vi "固件升级对话框.vi"() -> ()   [LabVIEW 2016, in "斯坦道通用流路CODmn.lvlib"]
uses:
  <vilib>/Utility/miscctls.llb/LVPointTypeDef.ctl
panel:
  in  "备份参数":bool
  in  "恢复参数":bool
  in  "关闭":bool
  in  "固件升级":bool
  in  "固件状态":bool
  out "结果字符串":string
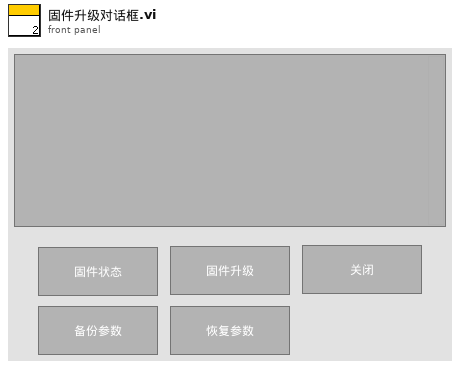
[diagram p1: front panel]
types:
  T1 = typedef "LVPointTypeDef.ctl" = cluster{"Horizontal":i16, "Vertical":i16}
  T2 = typedef "操作日志字段定义.ctl" = cluster{"时间":timestamp, "参数":string, "日志信息":string, "流程参数":string}
  T3 = cluster{"Value":u16, i32, i32, "公式":cluster{"X^2":dbl, "X":dbl, "b":dbl}, "error out":errorcluster}[][][]
  T4 = cluster{"Value":u16, "量程参数读取":cluster{"测量精度":u16, "检出限":dbl, "上限":dbl, "下限":dbl, "阈值（低->高）":dbl, "阈值（高->低）":dbl, "稀释度":dbl}, "error out":errorcluster}[]
  T5 = cluster{"试剂容量":cluster{"V1":sgl, "V2":sgl, "V3":sgl, "V4":sgl, "V5":sgl, "V6":sgl, "V7":sgl, "V8":sgl, "V9":sgl, "V10":sgl, "V11":sgl, "V12":sgl, "V9-1":sgl, "V9-2":sgl}, "error out":errorcluster}
  T6 = typedef "SingleStepTestV3.lvlib/SingleStepTestV3.lvclass/仪器版本.ctl" = enum16{"A版", "B版", "A1版"}
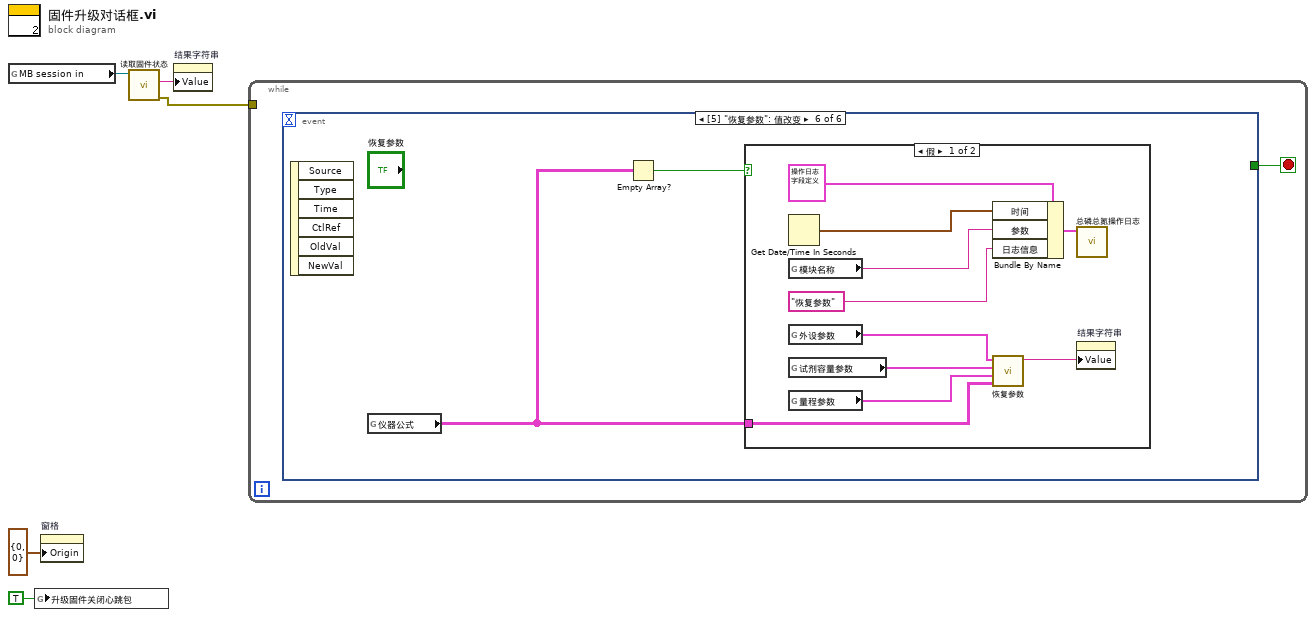
[diagram p0: block diagram]
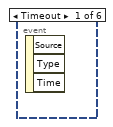
[diagram p2: hidden frame]
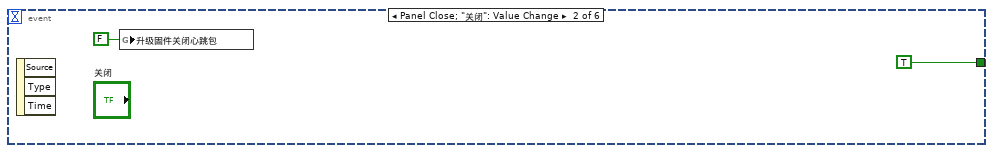
[diagram p3: hidden frame]
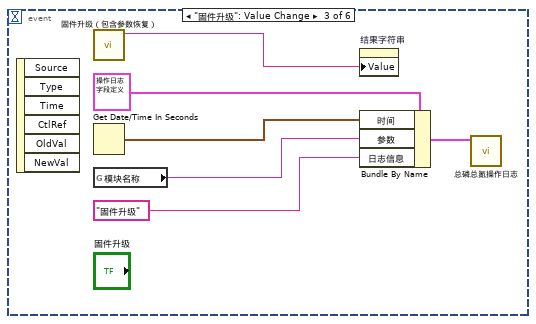
[diagram p4: hidden frame]
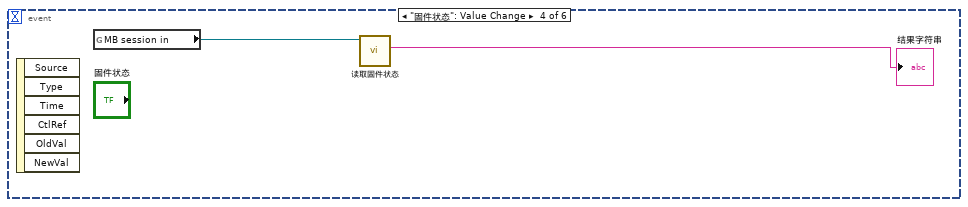
[diagram p5: hidden frame]
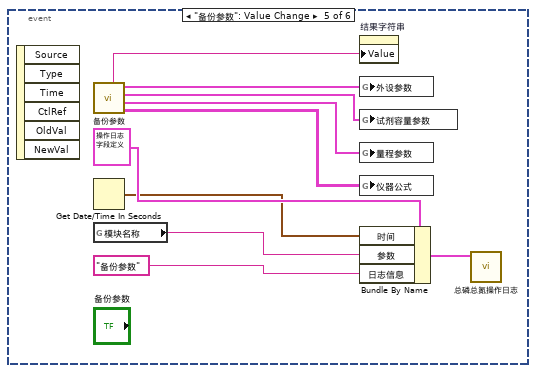
[diagram p6: hidden frame]
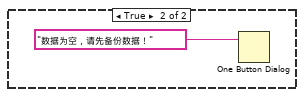
[diagram p7: hidden frame]
diagram:
  n1 = global read "VAR总磷总氮全局变量.vi" "MB session in"() -> (w4:refnum<class "MB_Master.lvclass">)
  n2 = global write "VAR总磷总氮全局变量.vi" "升级固件关闭心跳包"(TRUE ("升级固件关闭心跳包")) -> ()
  n3 = property on="窗格" class="Pane"("Origin"=T1 {"Horizontal"=0, "Vertical"=0} ("原点")) -> ()  [unwired: 2 in, 2 out]
  n4 = call "读取固件状态.vi"("MB session in"=w4) -> ("error out"=w3:errorcluster, "结果字符串"=w1:string)  [unwired: 7 in, 2 out]
  n5 = property on="结果字符串" class="Str"("Value"=w1) -> ()  [unwired: 2 in, 2 out]
  n6 = while {
    tunnel: w3 -> [_]
    stop <- w6 stop-if-true
    n7 = event shown="[5] \"恢复参数\": 值改变" {
      selector: _ -> [_ _ _ _ _ _]
      dyn-events: _ -> [_ _ _ _ _ _]
      timeout: _ -> [_ _ _ _ _ _]
      tunnel: [_ TRUE _ _ _ _] -> w6
      event Timeout {
        n8 = event-data() -> ()  [unwired: 1 in, 3 out]
      }
      event Panel Close; "关闭": Value Change {
        n9 = event-data() -> ()  [unwired: 1 in, 3 out]
        n10 = global write "VAR总磷总氮全局变量.vi" "升级固件关闭心跳包"(FALSE ("升级固件关闭心跳包")) -> ()
      }
      event "固件升级": Value Change {
        n11 = event-data() -> ()  [unwired: 1 in, 6 out]
        n12 = call "固件升级（包含参数恢复）.vi"() -> ("结果字符串"=w14:string)  [unwired: 11 in]
        n13 = Get Date/Time In Seconds() -> (seconds since 1Jan1904=w11:timestamp)
        n14 = global read "VAR总磷总氮全局变量.vi" "模块名称"() -> (w9:string)
        n15 = property on="结果字符串" class="Str"("Value"=w14) -> ()  [unwired: 2 in, 2 out]
        n16 = Bundle By Name(cluster=T2 {"时间"=timestamp(0 s since 1904-01-01), "参数"="", "日志信息"="", "流程参数"=""} ("data in"), "时间"=w11, "参数"=w9, "日志信息"="固件升级") -> (w12:T2)
        n17 = call "总磷总氮操作日志.vi"("data in"=w12) -> ()  [unwired: 10 in, 1 out]
      }
      event "固件状态": Value Change {
        n18 = event-data() -> ()  [unwired: 1 in, 6 out]
        n19 = global read "VAR总磷总氮全局变量.vi" "MB session in"() -> (w15:refnum<class "MB_Master.lvclass">)
        n20 = call "读取固件状态.vi"("MB session in"=w15) -> ("结果字符串"=→"结果字符串":string)  [unwired: 7 in, 3 out]
      }
      event "备份参数": Value Change {
        n21 = event-data() -> ()  [unwired: 1 in, 6 out]
        n22 = call "备份参数.vi"() -> ("仪器公式"=w23:T3, "量程参数"=w24:T4, "试剂容量参数"=w25:T5, "外设参数"=w26:cluster{"仪器版本":T6, "error out":errorcluster}, "备份结果"=w22:string)  [unwired: 7 in]
        n23 = Get Date/Time In Seconds() -> (seconds since 1Jan1904=w19:timestamp)
        n24 = global read "VAR总磷总氮全局变量.vi" "模块名称"() -> (w17:string)
        n25 = property on="结果字符串" class="Str"("Value"=w22) -> ()  [unwired: 2 in, 2 out]
        n26 = global write "VAR总磷总氮全局变量.vi" "外设参数"(w26) -> ()
        n27 = global write "VAR总磷总氮全局变量.vi" "试剂容量参数"(w25) -> ()
        n28 = global write "VAR总磷总氮全局变量.vi" "量程参数"(w24) -> ()
        n29 = global write "VAR总磷总氮全局变量.vi" "仪器公式"(w23) -> ()
        n30 = Bundle By Name(cluster=T2 {"时间"=timestamp(0 s since 1904-01-01), "参数"="", "日志信息"="", "流程参数"=""} ("data in"), "时间"=w19, "参数"=w17, "日志信息"="备份参数") -> (w20:T2)
        n31 = call "总磷总氮操作日志.vi"("data in"=w20) -> ()  [unwired: 10 in, 1 out]
      }
      event "恢复参数": Value Change {
        n32 = event-data() -> ()  [unwired: 1 in, 6 out]
        n33 = global read "VAR总磷总氮全局变量.vi" "仪器公式"() -> (w28:T3)
        n34 = Empty Array?(array=w28) -> (empty?=w27:bool)
        n35 = case shown="假" w27 {
          tunnel: w28 -> [w34 _]
          frame False {
            n36 = Get Date/Time In Seconds() -> (seconds since 1Jan1904=w31:timestamp)
            n37 = global read "VAR总磷总氮全局变量.vi" "模块名称"() -> (w29:string)
            n38 = global read "VAR总磷总氮全局变量.vi" "外设参数"() -> (w36:cluster{"仪器版本":T6, "error out":errorcluster})
            n39 = global read "VAR总磷总氮全局变量.vi" "试剂容量参数"() -> (w37:T5)
            n40 = global read "VAR总磷总氮全局变量.vi" "量程参数"() -> (w38:T4)
            n41 = Bundle By Name(cluster=T2 {"时间"=timestamp(0 s since 1904-01-01), "参数"="", "日志信息"="", "流程参数"=""} ("data in"), "时间"=w31, "参数"=w29, "日志信息"="恢复参数") -> (w32:T2)
            n42 = call "恢复参数.vi"("仪器公式"=w34, "量程参数"=w38, "试剂容量参数"=w37, "外设参数"=w36) -> ("恢复结果"=w35:string)  [unwired: 7 in]
            n43 = call "总磷总氮操作日志.vi"("data in"=w32) -> ()  [unwired: 10 in, 1 out]
            n44 = property on="结果字符串" class="Str"("Value"=w35) -> ()  [unwired: 2 in, 2 out]
          }
          frame True {
            n45 = One Button Dialog(message="数据为空，请先备份数据！" ("消息")) -> ()  [unwired: 1 in, 1 out]
          }
        }
      }
    }
  }
